vi "ArmGetTargetText.vi"() -> (1 "TargetGamePiece":string, 3 "TargetArmPosition":string)   [LabVIEW 2020]
uses:
  ArmGlobal.vi
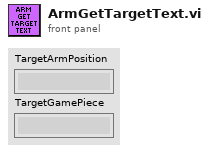
[diagram p1: front panel]
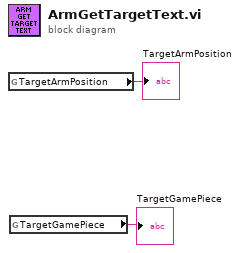
[diagram p0: block diagram]
diagram:
  n1 = global read "ArmGlobal.vi" "TargetArmPosition"() -> (→"TargetArmPosition":string)
  n2 = global read "ArmGlobal.vi" "TargetGamePiece"() -> (→"TargetGamePiece":string)
